vi "VI Tree.vi"   [LabVIEW 2013, in "Cal Inst.lvlib" / "California Instruments iX Series.lvlib"]
doc: "This is the instrument driver for the California Instruments iX Series. The VI Tree displays all the user-callable VIs of the instrument driver in an organized table."
uses:
  California Instruments iX Series.lvlib
  Data/Read Single Current Measurement.vi
  Data/Read Single Voltage Measurement.vi
panel:
  # "(c) 2009 National Instruments.  ALL RIGHTS RESERVED."
  # "SEE DIAGRAM\nFOR VI TREE."
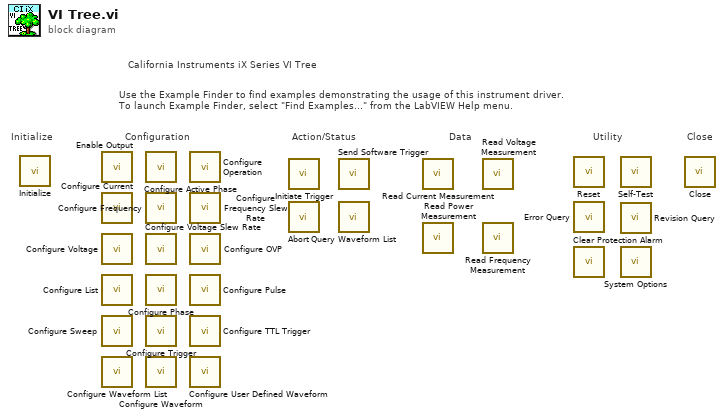
[diagram p0: block diagram]
diagram:
  # "California Instruments iX Series VI Tree"
  # "Use the Example Finder to find examples demonstrating the usage of this instrument driver.\nTo launch Example Finder, select \"Find Examples...\" from the LabVIEW Help menu."
  # "Configuration"
  # "Utility"
  # "Data"
  # "Action/Status"
  # "Close"
  # "Initialize"
  n1 = call "Initialize.vi"() -> ()  [unwired: 10 in, 2 out]
  n2 = call "Enable Output.vi"() -> ()  [unwired: 10 in, 2 out]
  n3 = call "Configure Current.vi"() -> ()  [unwired: 14 in, 2 out]
  n4 = call "Configure Voltage.vi"() -> ()  [unwired: 14 in, 2 out]
  n5 = call "Configure List.vi"() -> ()  [unwired: 10 in, 2 out]
  n6 = call "Configure Sweep.vi"() -> ()  [unwired: 10 in, 2 out]
  n7 = call "Configure Waveform List.vi"() -> ()  [unwired: 10 in, 2 out]
  n8 = call "Configure Active Phase.vi"() -> ()  [unwired: 14 in, 2 out]
  n9 = call "Configure Frequency.vi"() -> ()  [unwired: 14 in, 2 out]
  n10 = call "Configure Voltage Slew Rate.vi"() -> ()  [unwired: 14 in, 2 out]
  n11 = call "Configure Phase.vi"() -> ()  [unwired: 14 in, 2 out]
  n12 = call "Configure Trigger.vi"() -> ()  [unwired: 14 in, 2 out]
  n13 = call "Configure Waveform.vi"() -> ()  [unwired: 14 in, 2 out]
  n14 = call "Configure Operation.vi"() -> ()  [unwired: 10 in, 2 out]
  n15 = call "Configure Frequency Slew Rate.vi"() -> ()  [unwired: 14 in, 2 out]
  n16 = call "Configure OVP.vi"() -> ()  [unwired: 10 in, 2 out]
  n17 = call "Configure Pulse.vi"() -> ()  [unwired: 14 in, 2 out]
  n18 = call "Configure TTL Trigger.vi"() -> ()  [unwired: 14 in, 2 out]
  n19 = call "Configure User Defined Waveform.vi"() -> ()  [unwired: 14 in, 2 out]
  n20 = call "Initiate Trigger.vi"() -> ()  [unwired: 10 in, 2 out]
  n21 = call "Abort.vi"() -> ()  [unwired: 10 in, 2 out]
  n22 = call "Send Software Trigger.vi"() -> ()  [unwired: 10 in, 2 out]
  n23 = call "Query Waveform List.vi"() -> ()  [unwired: 9 in, 3 out]
  n24 = call-poly "Read Current Measurement.vi"() -> ()  [unwired: 9 in, 3 out]
  n25 = call "Read Power Measurement.vi"() -> ()  [unwired: 9 in, 3 out]
  n26 = call-poly "Read Voltage Measurement.vi"() -> ()  [unwired: 9 in, 3 out]
  n27 = call "Read Frequency Measurement.vi"() -> ()  [unwired: 9 in, 3 out]
  n28 = call "Reset.vi"() -> ()  [unwired: 10 in, 2 out]
  n29 = call "Error Query.vi"() -> ()  [unwired: 8 in, 4 out]
  n30 = call "Clear Protection Alarm.vi"() -> ()  [unwired: 10 in, 2 out]
  n31 = call "Self-Test.vi"() -> ()  [unwired: 8 in, 4 out]
  n32 = call "Revision Query.vi"() -> ()  [unwired: 8 in, 4 out]
  n33 = call "System Options.vi"() -> ()  [unwired: 14 in, 2 out]
  n34 = call "Close.vi"() -> ()  [unwired: 11 in, 1 out]
